vi "Wmeter Units.vi"(8 "error in":errorcluster, 10 "Combo Box":string(combo), 11 "WMeter":refnum<visa-resource-name>) -> (0 "error out":errorcluster, 3 "WMeter out":refnum<visa-resource-name>)   [LabVIEW 2012]
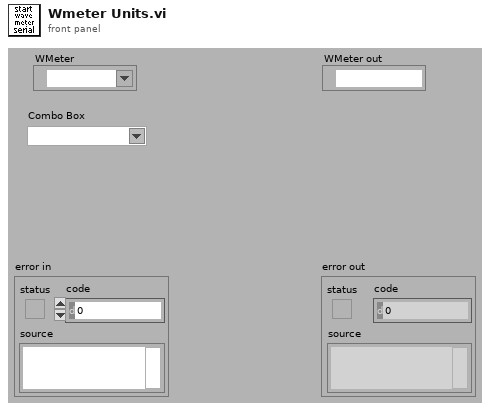
[diagram p1: front panel]
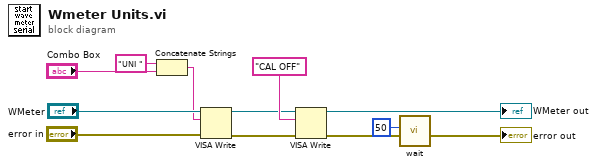
[diagram p0: block diagram]
diagram:
  n1 = Concatenate Strings("UNI " ("data"), "Combo Box") -> (w9:string)
  n2 = VISA Write(VISA resource name="WMeter", write buffer=w9, error in (no error)="error in") -> (VISA resource name out=w4:refnum<visa-resource-name>, error out=w5:errorcluster)  [unwired: 1 out]
  n3 = VISA Write(VISA resource name=w4, write buffer="CAL OFF" ("data"), error in (no error)=w5) -> (VISA resource name out=→"WMeter out":refnum<visa-resource-name>, error out=w7:errorcluster)  [unwired: 1 out]
  n4 = call "wait.vi"("error in (no error)"=w7, "ms to wait"=u32 50) -> ("error out (no error)"=→"error out":errorcluster)  [unwired: 7 in]
